vi "VARIABLES_GLOBAL.vi"() -> ()   [LabVIEW 2019]
panel:
  in  "TEMPERATURA":string
  in  "PH":string
  in  "HUMEDAD":string
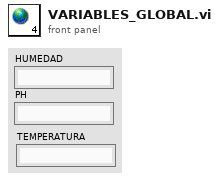
[diagram p1: front panel]
diagram:
